vi "FunctMgr.Pop and Return.vi"(8 "error in (no error)":errorcluster, 9 "Data":variant, 10 "Ret ID":string, 11 "FunctMgr in":refnum<class "FunctMgr.lvclass">) -> (0 "error out":errorcluster, 1 "Found":bool, 3 "FunctMgr out":refnum<class "FunctMgr.lvclass">)   [LabVIEW 2018, in "FunctMgr.lvclass"]
uses:
  FunctMgr.lvclass
  <vilib>/KATE/SeqMgr/SeqMgr.Ret Msg Info.ctl
  <vilib>/KATE/Queues/Q.Msg Return Info.ctl
  <vilib>/KATE/Queues/Q.Element.ctl
  FunctMgr.lvclass/FunctMgr.ctl
  <vilib>/KATE/Queues/Queue Utils.lvlib
  <vilib>/KATE/SeqMgr/SeqMgr.lvlib
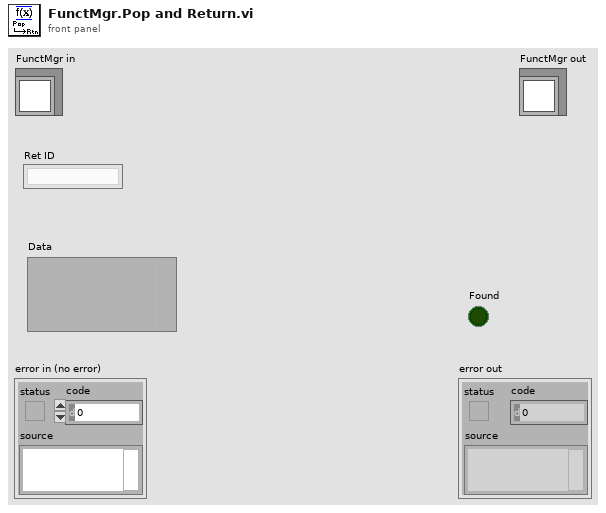
[diagram p1: front panel]
types:
  T1 = typedef "KATE_Lib.lvlib/SeqMgr.lvlib/SeqMgr.Ret Msg Info.ctl" = cluster{"ID":string, "Data":variant, "Ret Req":T2, "Error":errorcluster}
  T2 = typedef "KATE_Lib.lvlib/Queue Utils.lvlib/Q.Msg Return Info.ctl" = cluster{"Ret Q":refnum<queue>, "Ret Msg":T3, "SeqNum":i32}
  T3 = typedef "KATE_Lib.lvlib/Queue Utils.lvlib/Q.Element.ctl" = cluster{"Cmd":string, "Sub":string, "Data1":variant, "Data2":variant}
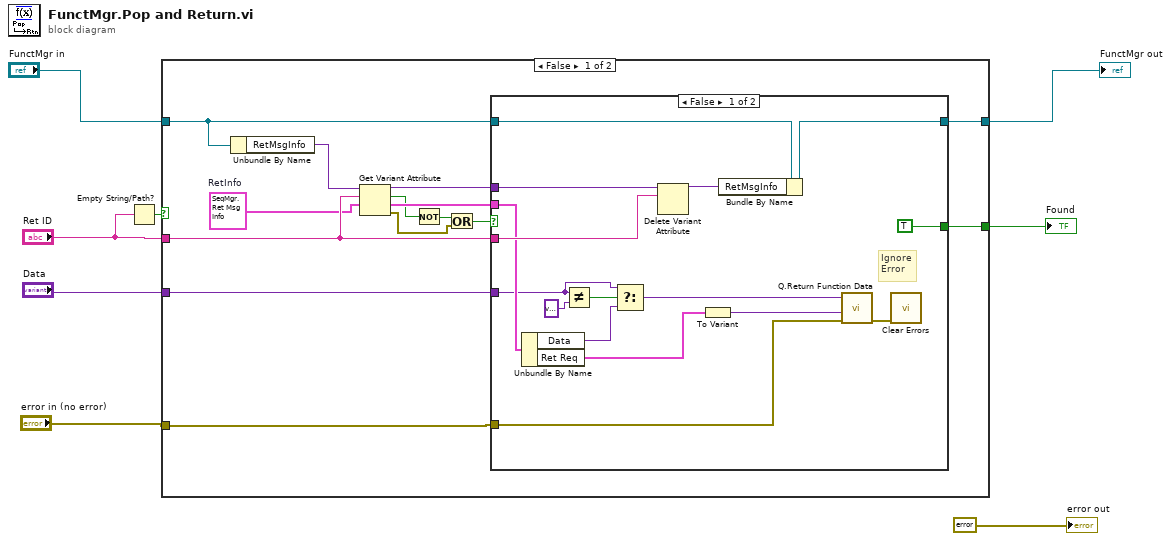
[diagram p0: block diagram]
diagram:
  n1 = Empty String/Path?(string/path="Ret ID") -> (empty?=w8:bool)
  n2 = case shown="False" w8 {
    tunnel: [w22 w40] -> w6
    tunnel: "FunctMgr in" -> [w21 w40]
    tunnel: "Ret ID" -> [w18 _]
    tunnel: [w12 _] -> w5
    tunnel: "Data" -> [w10 _]
    tunnel: "error in (no error)" -> [w9 _]
    frame False {
      w11 = T1 {"ID"="", "Data"=variant, "Ret Req"={"Ret Q"=refnum, "Ret Msg"={"Cmd"="", "Sub"="", "Data1"=variant, "Data2"=variant}, "SeqNum"=0}, "Error"={"status"=FALSE, "code"=0, "source"=""}}  # RetInfo
      n3 = Unbundle By Name(w21) -> ("RetMsgInfo"=w20:variant)
      n4 = Get Variant Attribute(Variant=w20, name=w18, default value (empty Variant)=w11) -> (duplicate Variant=w19:variant, found=w16:bool, value=w17:T1, error out=w14:errorcluster)  [unwired: 1 in]
      n5 = Not(x=w16) -> (.not. x?=w15:bool)
      n6 = Or(x=w15, y=w14) -> (x .or. y?=w13:bool)
      n7 = case shown="False" w13 {
        tunnel: [w38 w39] -> w22
        tunnel: w21 -> [w37 w39]
        tunnel: w19 -> [w36 _]
        tunnel: w18 -> [w35 _]
        tunnel: w17 -> [w32 _]
        tunnel: [TRUE _] -> w12
        tunnel: w9 -> [w29 _]
        tunnel: w10 -> [w25 _]
        frame False {
          # "Ignore\nError"
          n8 = Unbundle By Name(w32) -> ("Data"=w24:variant, "Ret Req"=w28:T2)
          n9 = Not Equal?(x=w25, y=variant) -> (x != y?=w26:bool)
          n10 = Select(t=w25, s=w26, f=w24) -> (s? t:f=w23:variant)
          n11 = Delete Variant Attribute(6:w35, 7:w36) -> (3:w34:variant)  [unwired: 1 in, 2 out]
          n12 = To Variant(anything=w28) -> (Variant=w31:variant)
          n13 = Bundle By Name(cluster=w37, "RetMsgInfo"=w34) -> (w38:refnum<class "FunctMgr.lvclass">)
          n14 = call <vilib>:"Q.Return Function Data.vi"("error in"=w29, "Data2"=w31, "Ret Data"=w23) -> ("error out"=w30:errorcluster)  [unwired: 8 in]
          n15 = call <vilib>:"Clear Errors.vi"("error in (no error)"=w30) -> ()  [unwired: 5 in, 2 out]
        }
        frame True {
          # "Do nothing\nError or not found"
        }
      }
    }
    frame True {
      # "Do nothing\nEmpty ID"
    }
  }
  "FunctMgr out" <- w6
  "Found" <- w5
  "error out" <- errorcluster {"status"=FALSE, "code"=0, "source"=""} ("error constant")
